vi "Kinesis - KNA - Set Circle Diameter.vi"() -> ()   [LabVIEW 2012]
doc: "Shows how to set and get the NanoTrak circle diameter."
uses:
  C:/Users/bhallewell/Desktop/Kinesis_with_LabVIEW_Examples_LV12_v1/Thorlabs.MotionControl.Controls.dll
  Thorlabs.MotionControl.Controls.dll
  C:/Users/bhallewell/Desktop/Kinesis_with_LabVIEW_Examples_LV12_v1/Thorlabs.MotionControl.KCube.NanoTrakCLI.dll
  Thorlabs.MotionControl.KCube.NanoTrakCLI.dll
panel:
  in  "?":bool
  in  "?":dbl
  out "?":dbl
  in  "?":bool
  in  "?":bool
  in  "SerialNumber":string
  in  "KCubeNanoTrakControl":refnum<k24>(container)
  # "Notes:"
  # "- Ensure that the appropriate .DLLs are copied into your Project Folder. Check that the correct bit type are used depending on your version of LabVIEW\ni.e. 32-bit or 64-bit.\n\n\n\n\n\n\n\n\n\n\n\n\n\n\n- Open the example VI through the LabVIEW Project Explorer to correctly load the User Interface from Thorlabs.MotionControl.Controls.dll."
  # "Thorlabs Hardware: KNA - K-Cube Nanotrak Controller\nhttps://www.thorlabs.com/newgrouppage9.cfm?objectgroup_id=2877"
  # "This VI will enable you to run the Kinesis Device panel for KNA-nnn devices. \nYou will also be able to set the Scan Circle Diameter in the range of 0 to 10 NT Units.\n\nInstructions:\n1. Connect your KNA-nnn device to your PC via USB & power your device.\n2. Enter the serial number of the controller into the SerialNumber box below.\n3. Run the VI from the LabVIEW Toolbar.\n4. Enter a circle diameter (0 to 10 NT units) & click 'SET DIAMETER'.\n5. To close the program click 'END PROGRAM'."
  # "Example Image of .NET Controller - VI opened via Project Explorer/ not opened via Project Explorer"
  # "VI Not Opened via Project Explorer"
  # "VI Opened via Project Explorer"
  # "- To explore the range of methods available, please visit the .NET API, included with your Kinesis software.\n\n- For tips on building your own VIs with Thorlabs Motion Control Hardware, please see our LabVIEW Guide here.\nhttps://www.thorlabs.com/newgrouppage9.cfm?objectgroup_id=10285"
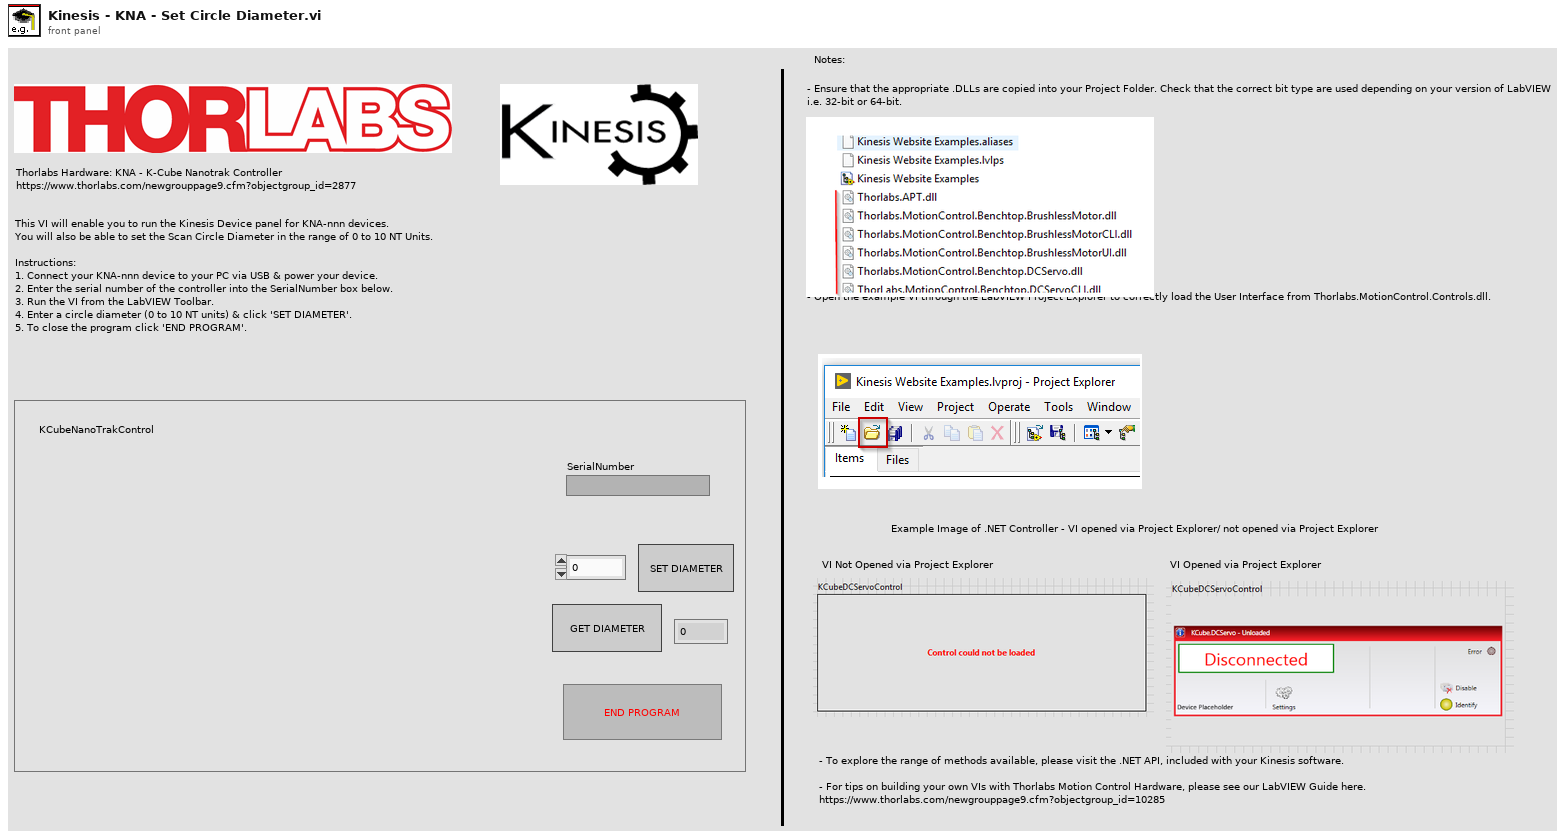
[diagram p1: front panel]
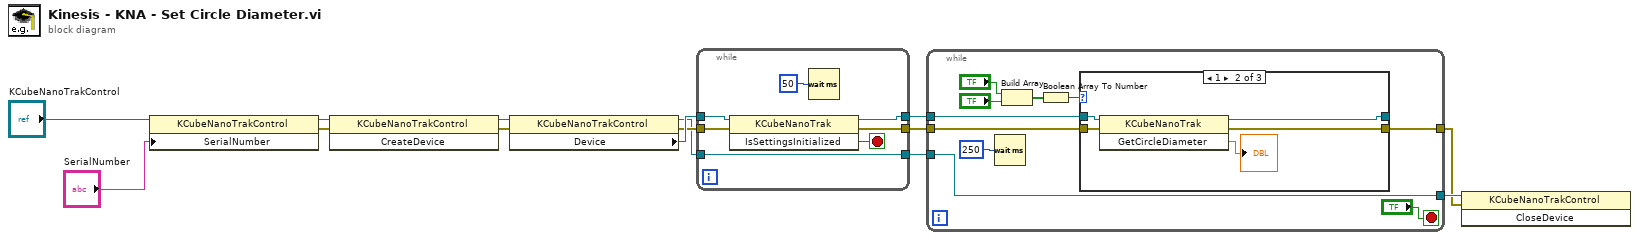
[diagram p0: block diagram]
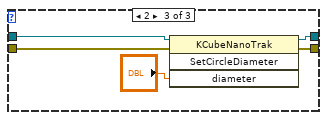
[diagram p3: hidden frame]
diagram:
  n1 = property class="KCubeNanoTrakControl"(reference="KCubeNanoTrakControl", "SerialNumber"="SerialNumber") -> (reference out=w12:refnum<k24>, error out=w11:errorcluster)  [unwired: 1 in]
  n2 = invoke class="KCubeNanoTrakControl" method="CreateDevice"(reference=w12, error in=w11) -> (reference out=w14:refnum<k24>, error out=w13:errorcluster)  [unwired: 1 in, 1 out]
  n3 = property class="KCubeNanoTrakControl"(reference=w14, error in=w13) -> (reference out=w2:refnum<k24>, error out=w6:errorcluster, "Device"=w8:refnum<k24>)
  n4 = while {
    tunnel: w8 -> [w19]
    tunnel: [w18] -> w7
    tunnel: w6 -> [w17]
    tunnel: [w16] -> w5
    tunnel: [w15] -> w3
    tunnel: w2 -> [w15]
    stop <- w21 stop-if-true
    n5 = invoke class="KCubeNanoTrak" method="IsSettingsInitialized"(reference=w19, error in=w17) -> (reference out=w18:refnum<k24>, error out=w16:errorcluster, "IsSettingsInitialized"=w21:bool)  [unwired: 1 in]
    n6 = Wait (ms)(milliseconds to wait=u32 50) -> ()  [unwired: 1 out]
  }
  n7 = while {
    tunnel: w7 -> [w27]
    tunnel: w5 -> [w25]
    tunnel: [w23] -> w4
    tunnel: w3 -> [w23]
    tunnel: [w22] -> w1
    stop <- "?" stop-if-true
    n8 = Wait (ms)(milliseconds to wait=u32 250) -> ()  [unwired: 1 out]
    n9 = Build Array("?", "?") -> (w29:bool[])
    n10 = Boolean Array To Number(Boolean array=w29) -> (number=w28:u32)
    n11 = case shown="1" w28 {
      tunnel: [w33 w37 w42] -> _
      tunnel: w27 -> [w33 w38 w43]
      tunnel: w25 -> [w32 w35 w40]
      tunnel: [w32 w34 w39] -> w22
      frame 0, Default {
      }
      frame 1 {
        n12 = invoke class="KCubeNanoTrak" method="GetCircleDiameter"(reference=w38, error in=w35) -> (reference out=w37:refnum<k24>, error out=w34:errorcluster, "GetCircleDiameter"=→"?":dbl)  [unwired: 1 in]
      }
      frame 2 {
        n13 = invoke class="KCubeNanoTrak" method="SetCircleDiameter"(reference=w43, error in=w40, "diameter"="?") -> (reference out=w42:refnum<k24>, error out=w39:errorcluster)  [unwired: 1 in, 2 out]
      }
    }
  }
  n14 = invoke class="KCubeNanoTrakControl" method="CloseDevice"(reference=w4, error in=w1) -> ()  [unwired: 1 in, 3 out]
